vi "Polar To Complex - RM,R.vi"(1 "Argument Scalar Q":dbl, 2 "Modulus r":T2) -> (0 "Complex Matrix r*e^iQ":T1)   [LabVIEW 2017, in "NI_Matrix.lvlib"]
doc: "Creates a complex number from two values in polar notation."
uses:
  <vilib>/Analysis/Matrix/NI_Matrix.lvlib
  <vilib>/Analysis/Matrix/Datatypes/RealMatrix.ctl
  <vilib>/Analysis/Matrix/Datatypes/ComplexMatrix.ctl
  <vilib>/Analysis/Matrix/Numeric/Conversions/Array To Matrix - CA2.vi
  <vilib>/Analysis/Matrix/Numeric/Conversions/Matrix To Array - RM.vi
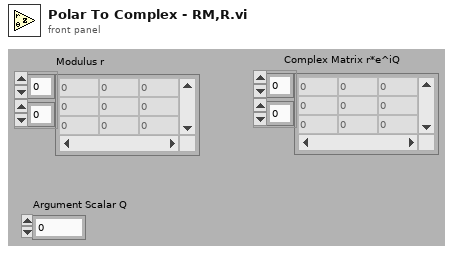
[diagram p1: front panel]
types:
  T1 = typedef "NI_Matrix.lvlib/ComplexMatrix.ctl" = cdb[][]
  T2 = typedef "NI_Matrix.lvlib/RealMatrix.ctl" = dbl[][]
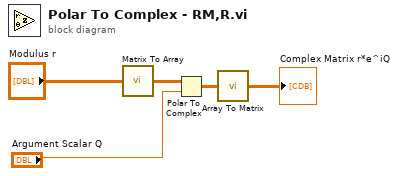
[diagram p0: block diagram]
diagram:
  n1 = call-poly <vilib>:"Matrix To Array.vi"("Real Matrix"="Modulus r") -> ("Real 2D Array"=w4:dbl[][])
  n2 = Polar To Complex(1:"Argument Scalar Q", 2:w4) -> (0:w2:cdb[][])
  n3 = call-poly <vilib>:"Array To Matrix.vi"("Complex 2D Array"=w2) -> ("Complex Matrix"=→"Complex Matrix r*e^iQ":T1)
